vi "BlueSimpleReachTask.vi"() -> ()   [LabVIEW 2010]
uses:
  Controls/Bits to Write.ctl
panel:
  in  "Catch probability":i32 min=0 max=100 step=1
  out "Catch Trial?":bool
  in  "Catch Trial":bool
  out "DO Task":refnum<k21>="BlueSimple_DO_All"
  out "DI Task":refnum<k21>="BlueSimple_DI"
  out "Exp correct":i32
  out "Record flag":bool
  in  "Recenter motor":bool
  in  "Override bumps":bool
  in  "Start bump timer?":bool
  in  "Trial type":u16(ring) items=["Allflash/sensory", "Precue/memory"]
  in  "DBS On?":bool
  in  "Home+target OK?":bool
  out "Exp reset":bool
  out "target set #":i32
  in  "duration (s)":dbl=0.18 format="%.4f"
  in  "Inter-pulse delay":cluster{"Fix":dbl, "Rnd":dbl}={"Fix"=0.0, "Rnd"=1.5} {"Rnd" format="%.4f"; "Fix" format="%_4g"}
  in  "Autofeed?":bool
  out "Just initialized\nhold loop?":bool
  in  "Home reward?":bool
  in  "Home reward":cluster{"Fix":dbl, "Rnd":dbl} {"Rnd" format="%.4f"; "Fix" format="%_4g"}
  in  "Override 4":bool caption="Override 1"
  in  "Override 3":bool caption="Override 1"
  in  "Override 2":bool=TRUE caption="Override 1"
  in  "Override 1":bool=TRUE
  in  "LED lines":T1={"LED1"=1, "LED2"=2, "LED3"=3, "LED4"=4}
  in  "LED1":i16=5
  in  "LED2":i16=6
  in  "LED3":i16=7
  in  "LED4":i16=8
  in  "Bump Parameters":T2={"Distance (deg)"=2.0, "Travel time (ms)"=500.0} {"Travel time (ms)" min=0.1 max=10000.0; "Distance (deg)" min=0.1}
  in  "Bump delay":cluster{"Fix":dbl, "Rnd":dbl}={"Fix"=2.0, "Rnd"=8.0} {"Rnd" format="%.4f"; "Fix" format="%_4g"}
  in  "Sine parameters":T3={"Frequency"=1.0, "Degrees\npk-pk"=8.0, "Cycles"=10000} {"Degrees\npk-pk" min=0.1 max=120.0; "Frequency" min=0.001 format="%#_4g"}
  in  "Home":bool
  in  "Bumps":bool
  in  "Sines?":bool
  out "target set size":i32
  out "# target sets":u16
  in  "# Cycles":i16=20
  out "Instruct duration":dbl format="%.4f"
  out "Pre-I hold":dbl format="%.4f"
  out "Touching target\nlast time?":bool
  in  "Rand/Seq?":bool=TRUE
  in  "Target set":i16[](array[ring]) items=["1", "2", "3", "4"]
  in  "Block":T4(array[cluster])=array[6501 elements]
  in  "Settings In":T5={"Pre-I hold"={"Fixed (s)"=0.5, "Random (s)"=0.5}, "LED I duration"={"Fixed (s)"=0.5, "Random (s)"=0.0}, "All Flash?"=FALSE, "Pre-cue brightness"=0, "Post-I hold"={"Fixed (s)"=0.7, "Random (s)"=0.3}, "Post-I \nbounce-off"={"Fixed (s)"=0.3, "Random (s)"=0.0}, "Capture timeout"={"Fixed (s)"=1.5, "Random (s)"=0.0}, "Tone duration"={"Fixed (s)"=0.5, "Random (s)"=0.0}, "LED C duration"={"Fixed (s)"=0.5, "Random (s)"=0.0}, "Cue brightness"=0, "Hold duration"={"Fixed (s)"=0.3, "Random (s)"=0.0}, "Allowed\nbounce-off"={"Fixed (s)"=0.2, "Random (s)"=0.0}, "Post-capture brightness"=0, "Reward duration"={"Fixed (s)"=0.7, "Random (s)"=0.0}, "Intertrial interval"={"Fixed (s)"=0.5, "Random (s)"=0.0}, "Persistent Mode?"=FALSE, "Error bong?"=TRUE, "Critter"=0, "Blocks"=[], "Target set"=[], "Rand/Seq?"=TRUE, "Trial type"=0, "Sines?"=FALSE, "Bumps"=FALSE, "Sine parameters"={"Frequency"=0.25, "Degrees\npk-pk"=6.0, "Cycles"=10000}, "Bump timing"={"Fix"=2.0, "Rnd"=8.0}, "Bump Parameters"={"Distance (deg)"=2.0, "Travel time (ms)"=500.0}, "DBS On?"=FALSE, "Home reward?"=FALSE, "Home+target OK?"=FALSE} {"Bump Parameters"."Travel time (ms)" min=0.1 max=10000.0; "Bump Parameters"."Distance (deg)" min=0.1; "Bump timing"."Rnd" format="%.4f"; "Bump timing"."Fix" format="%_4g"; "Sine parameters"."Degrees\npk-pk" min=0.1 max=120.0; "Sine parameters"."Frequency" min=0.001 format="%#_4g"; "Trial type" items=["Allflash/sensory", "Precue/memory"]; "Target set" items=["1", "2", "3", "4"]; "Critter" items=["Mojo", "Smokey"]; "Post-I \nbounce-off"."Random (s)" format="%.4f"; "Post-I \nbounce-off"."Fixed (s)" format="%_4g"; "Allowed\nbounce-off"."Random (s)" format="%.4f"; "Allowed\nbounce-off"."Fixed (s)" format="%_4g"; "LED C duration"."Random (s)" format="%.4f"; "LED C duration"."Fixed (s)" format="%.4f"; "Capture timeout"."Random (s)" format="%.4f"; "Capture timeout"."Fixed (s)" format="%.4f"; "Post-I hold"."Random (s)" format="%.4f"; "Post-I hold"."Fixed (s)" format="%.4f"; "Hold duration"."Random (s)" format="%.4f"; "Hold duration"."Fixed (s)" format="%_4g"; "Intertrial interval"."Random (s)" format="%.4f"; "Intertrial interval"."Fixed (s)" format="%.4f"; "Reward duration"."Random (s)" format="%.4f"; "Reward duration"."Fixed (s)" format="%.4f"; "LED I duration"."Random (s)" format="%.4f"; "LED I duration"."Fixed (s)" format="%.4f"; "Tone duration"."Random (s)" format="%.4f"; "Tone duration"."Fixed (s)" format="%.4f"; "Pre-I hold"."Random (s)" format="%.4f"; "Pre-I hold"."Fixed (s)" format="%_4g"}
  in  "pause":bool
  out "Assign settings":bool
  out "current path":path
  out "next trial path":path
  in  "Critter":u16(ring) items=["Mojo", "Smokey", "Blue", "Odo", "Monk 5", "Monk 6", "Monk 7", "Monk 8", "Monk 9", "Monk 10"]
  out "Total incorrect":i32
  in  "Write Settings":bool
  in  "Read Settings":bool
  in  "All Flash?":bool
  in  "Post-capture brightness":i16 caption="Brightness"
  in  "Cue brightness":i16=6 caption="Brightness"
  in  "Pre-cue brightness":i16 caption="Brightness"
  out "Total correct":i32
  out "Total %":dbl
  out "Total trials":i32
  in  "Error\nbong?":bool=TRUE
  out "TS Home":bool
  out "TS 4":bool
  out "TS 3":bool
  out "TS 2":bool
  out "TS 1":bool
  out "Waveform Chart":T6(graph)
  out "Block trials":i32
  out "Block %":dbl
  in  "Reset\ncounters":bool
  in  "Post-I \nbounce-off":cluster{"Fix":dbl, "Rnd":dbl}={"Fix"=0.3, "Rnd"=0.0} caption="Allowed\nbounce-off" {"Rnd" format="%.4f"; "Fix" format="%_4g"}
  out "Exp trials":i32
  out "Exp %":dbl
  in  "Touch lines":T7={"Home touch"=0, "Touch 1"=1, "Touch 2"=2, "Touch 3"=3, "Touch 4"=4}
  out "Current stage":T8(ring)
  in  "Allowed\nbounce-off":cluster{"Fix":dbl, "Rnd":dbl}={"Fix"=0.2, "Rnd"=0.0} {"Rnd" format="%.4f"; "Fix" format="%_4g"}
  in  "LED C duration":cluster{"Fix":dbl, "Rnd":dbl}={"Fix"=0.5, "Rnd"=0.0} caption="LED duration" {"Rnd" format="%.4f"; "Fix" format="%.4f"}
  in  "Capture timeout":cluster{"Fix":dbl, "Rnd":dbl}={"Fix"=1.5, "Rnd"=0.0} caption="Response time" {"Rnd" format="%.4f"; "Fix" format="%.4f"}
  in  "Post-I hold":cluster{"Fix":dbl, "Rnd":dbl}={"Fix"=0.5, "Rnd"=0.5} {"Rnd" format="%.4f"; "Fix" format="%.4f"}
  out "Last trial successful?":bool
  in  "Persistent\n Mode?":bool
  in  "Touch 4":i16=4
  in  "Touch 3":i16=3
  in  "Touch 2":i16=2
  in  "Touch 1":i16=1
  in  "Home touch":i16
  in  "Hold duration":cluster{"Fix":dbl, "Rnd":dbl}={"Fix"=0.3, "Rnd"=0.0} {"Rnd" format="%.4f"; "Fix" format="%_4g"}
  out "Target":i16
  in  "stop":bool
  in  "device":i16=1
  in  "line direction map":i32=2147483616 format="%.0b"
  out "DIGIO task ID":u32 format="%.0x"
  out "error out":errorcluster
  in  "Intertrial interval":cluster{"Fix":dbl, "Rnd":dbl}={"Fix"=0.5, "Rnd"=0.0} {"Rnd" format="%.4f"; "Fix" format="%.4f"}
  in  "Reward duration":cluster{"Fix":dbl, "Rnd":dbl}={"Fix"=0.7, "Rnd"=0.0} {"Rnd" format="%.4f"; "Fix" format="%.4f"}
  in  "LED I duration":cluster{"Fix":dbl, "Rnd":dbl}={"Fix"=0.5, "Rnd"=0.0} caption="LED duration" {"Rnd" format="%.4f"; "Fix" format="%.4f"}
  in  "Tone duration":cluster{"Fix":dbl, "Rnd":dbl}={"Fix"=0.5, "Rnd"=0.0} {"Rnd" format="%.4f"; "Fix" format="%.4f"}
  in  "Pre-I hold":cluster{"Fix":dbl, "Rnd":dbl}={"Fix"=0.5, "Rnd"=0.5} {"Rnd" format="%.4f"; "Fix" format="%_4g"}
  # "Auto-feed"
  # "DBS"
  # "Pre-\ninstruction\nhold"
  # "Post-\ninstruction\nhold"
  # "Instruction"
  # "Target capture"
  # "Target hold"
  # "Reward"
  # "Intertrial"
  # "Motor"
  # "Override"
  # "+"
  # "+"
  # "+"
  # "Pre-\ninstruction\nhold"
  # "Instruction"
  # "Post-\ninstruction\nhold"
  # "Target capture"
  # "Target hold"
  # "Reward"
  # "Intertrial"
  # "+"
  # "+"
  # "+"
  # "+"
  # "+"
  # "+"
  # "+"
  # "+"
  # "+"
  # "+"
  # "+"
  # "+"
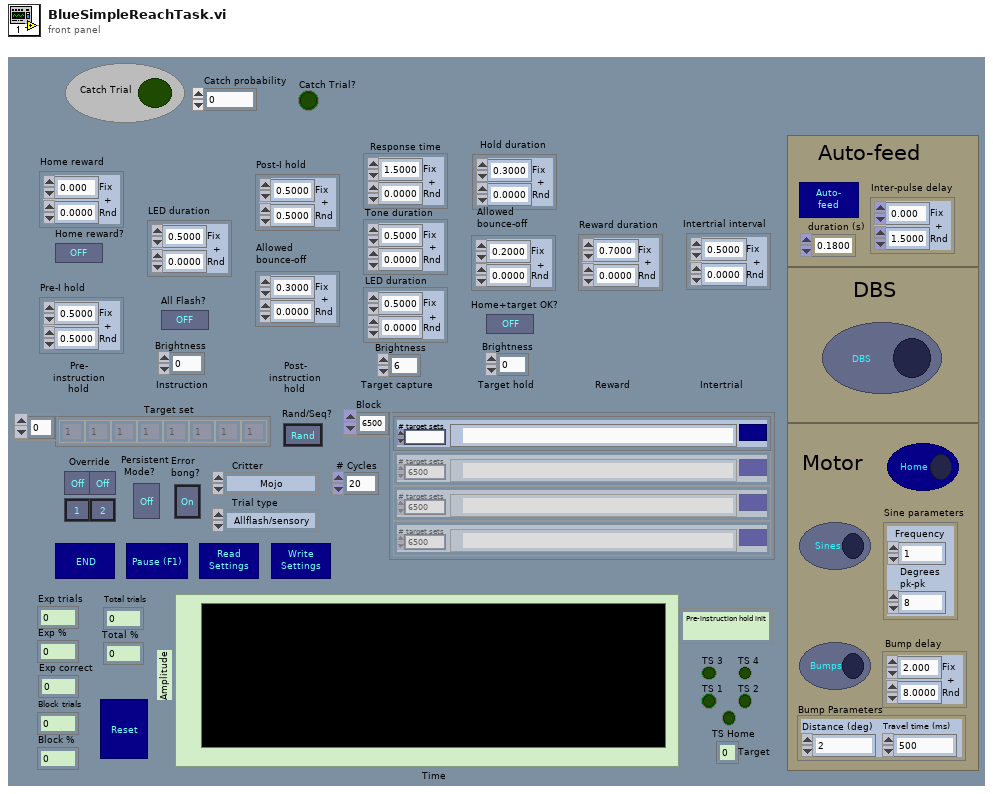
[diagram p1: front panel]
types:
  T1 = cluster{"LED1":i16, "LED2":i16, "LED3":i16, "LED4":i16}
  T2 = cluster{"Distance (deg)":dbl, "Travel time (ms)":dbl}
  T3 = cluster{"Frequency":dbl, "Degrees\npk-pk":dbl, "Cycles":i16}
  T4 = cluster{"Settings file":path, "# target sets":u16}[]
  T5 = cluster{"Pre-I hold":cluster{"Fixed (s)":dbl, "Random (s)":dbl}, "LED I duration":cluster{"Fixed (s)":dbl, "Random (s)":dbl}, "All Flash?":bool, "Pre-cue brightness":i16, "Post-I hold":cluster{"Fixed (s)":dbl, "Random (s)":dbl}, "Post-I \nbounce-off":cluster{"Fixed (s)":dbl, "Random (s)":dbl}, "Capture timeout":cluster{"Fixed (s)":dbl, "Random (s)":dbl}, "Tone duration":cluster{"Fixed (s)":dbl, "Random (s)":dbl}, "LED C duration":cluster{"Fixed (s)":dbl, "Random (s)":dbl}, "Cue brightness":i16, "Hold duration":cluster{"Fixed (s)":dbl, "Random (s)":dbl}, "Allowed\nbounce-off":cluster{"Fixed (s)":dbl, "Random (s)":dbl}, "Post-capture brightness":i16, "Reward duration":cluster{"Fixed (s)":dbl, "Random (s)":dbl}, "Intertrial interval":cluster{"Fixed (s)":dbl, "Random (s)":dbl}, "Persistent Mode?":bool, "Error bong?":bool, "Critter":u16, "Blocks":cluster{"Settings file":path, "# target sets":dbl}[], "Target set":i16[], "Rand/Seq?":bool, "Trial type":u16, "Sines?":bool, "Bumps":bool, "Sine parameters":cluster{"Frequency":dbl, "Degrees\npk-pk":dbl, "Cycles":i16}, "Bump timing":cluster{"Fix":dbl, "Rnd":dbl}, "Bump Parameters":cluster{"Distance (deg)":dbl, "Travel time (ms)":dbl}, "DBS On?":bool, "Home reward?":bool, "Home+target OK?":bool}
  T6 = cluster{"Segment Percentage":dbl, "Total % correct":dbl}
  T7 = cluster{"Home touch":i16, "Touch 1":i16, "Touch 2":i16, "Touch 3":i16, "Touch 4":i16}
  T8 = enum16{"Pre-instruction hold init", "Pre-instruction hold", "Instruction init", "Instruction", "Post-instruction hold init", "Post-instruction hold", "Target capture init", "Target capture", "Target hold init", "Target hold", "Reward stage", "Intertrial"}
  T9 = typedef "Bits to Write.ctl" = enum16{"LED 1 on", "LED 1 off", "LED 2 on", "LED 2 off", "LED 3 on", "LED 3 off", "LED 4 on", "LED 4 off", "All LEDs on", "All LEDs off", "In trial on", "In trial off", "Buzzer on", "Buzzer off", "Reward on", "Reward off", "Target number", "Trial type preQ on", "Trial type preQ off", "Error on", "Error off", "Trial number", "DBS on", "DBS off", "Sine on", "Sine off", "All Bits On", "All Bits Off", "Init", "Specify mask/pattern"}
  T10 = enum16{"Reset", "Increment", "Reset for exp", "Initialize"}
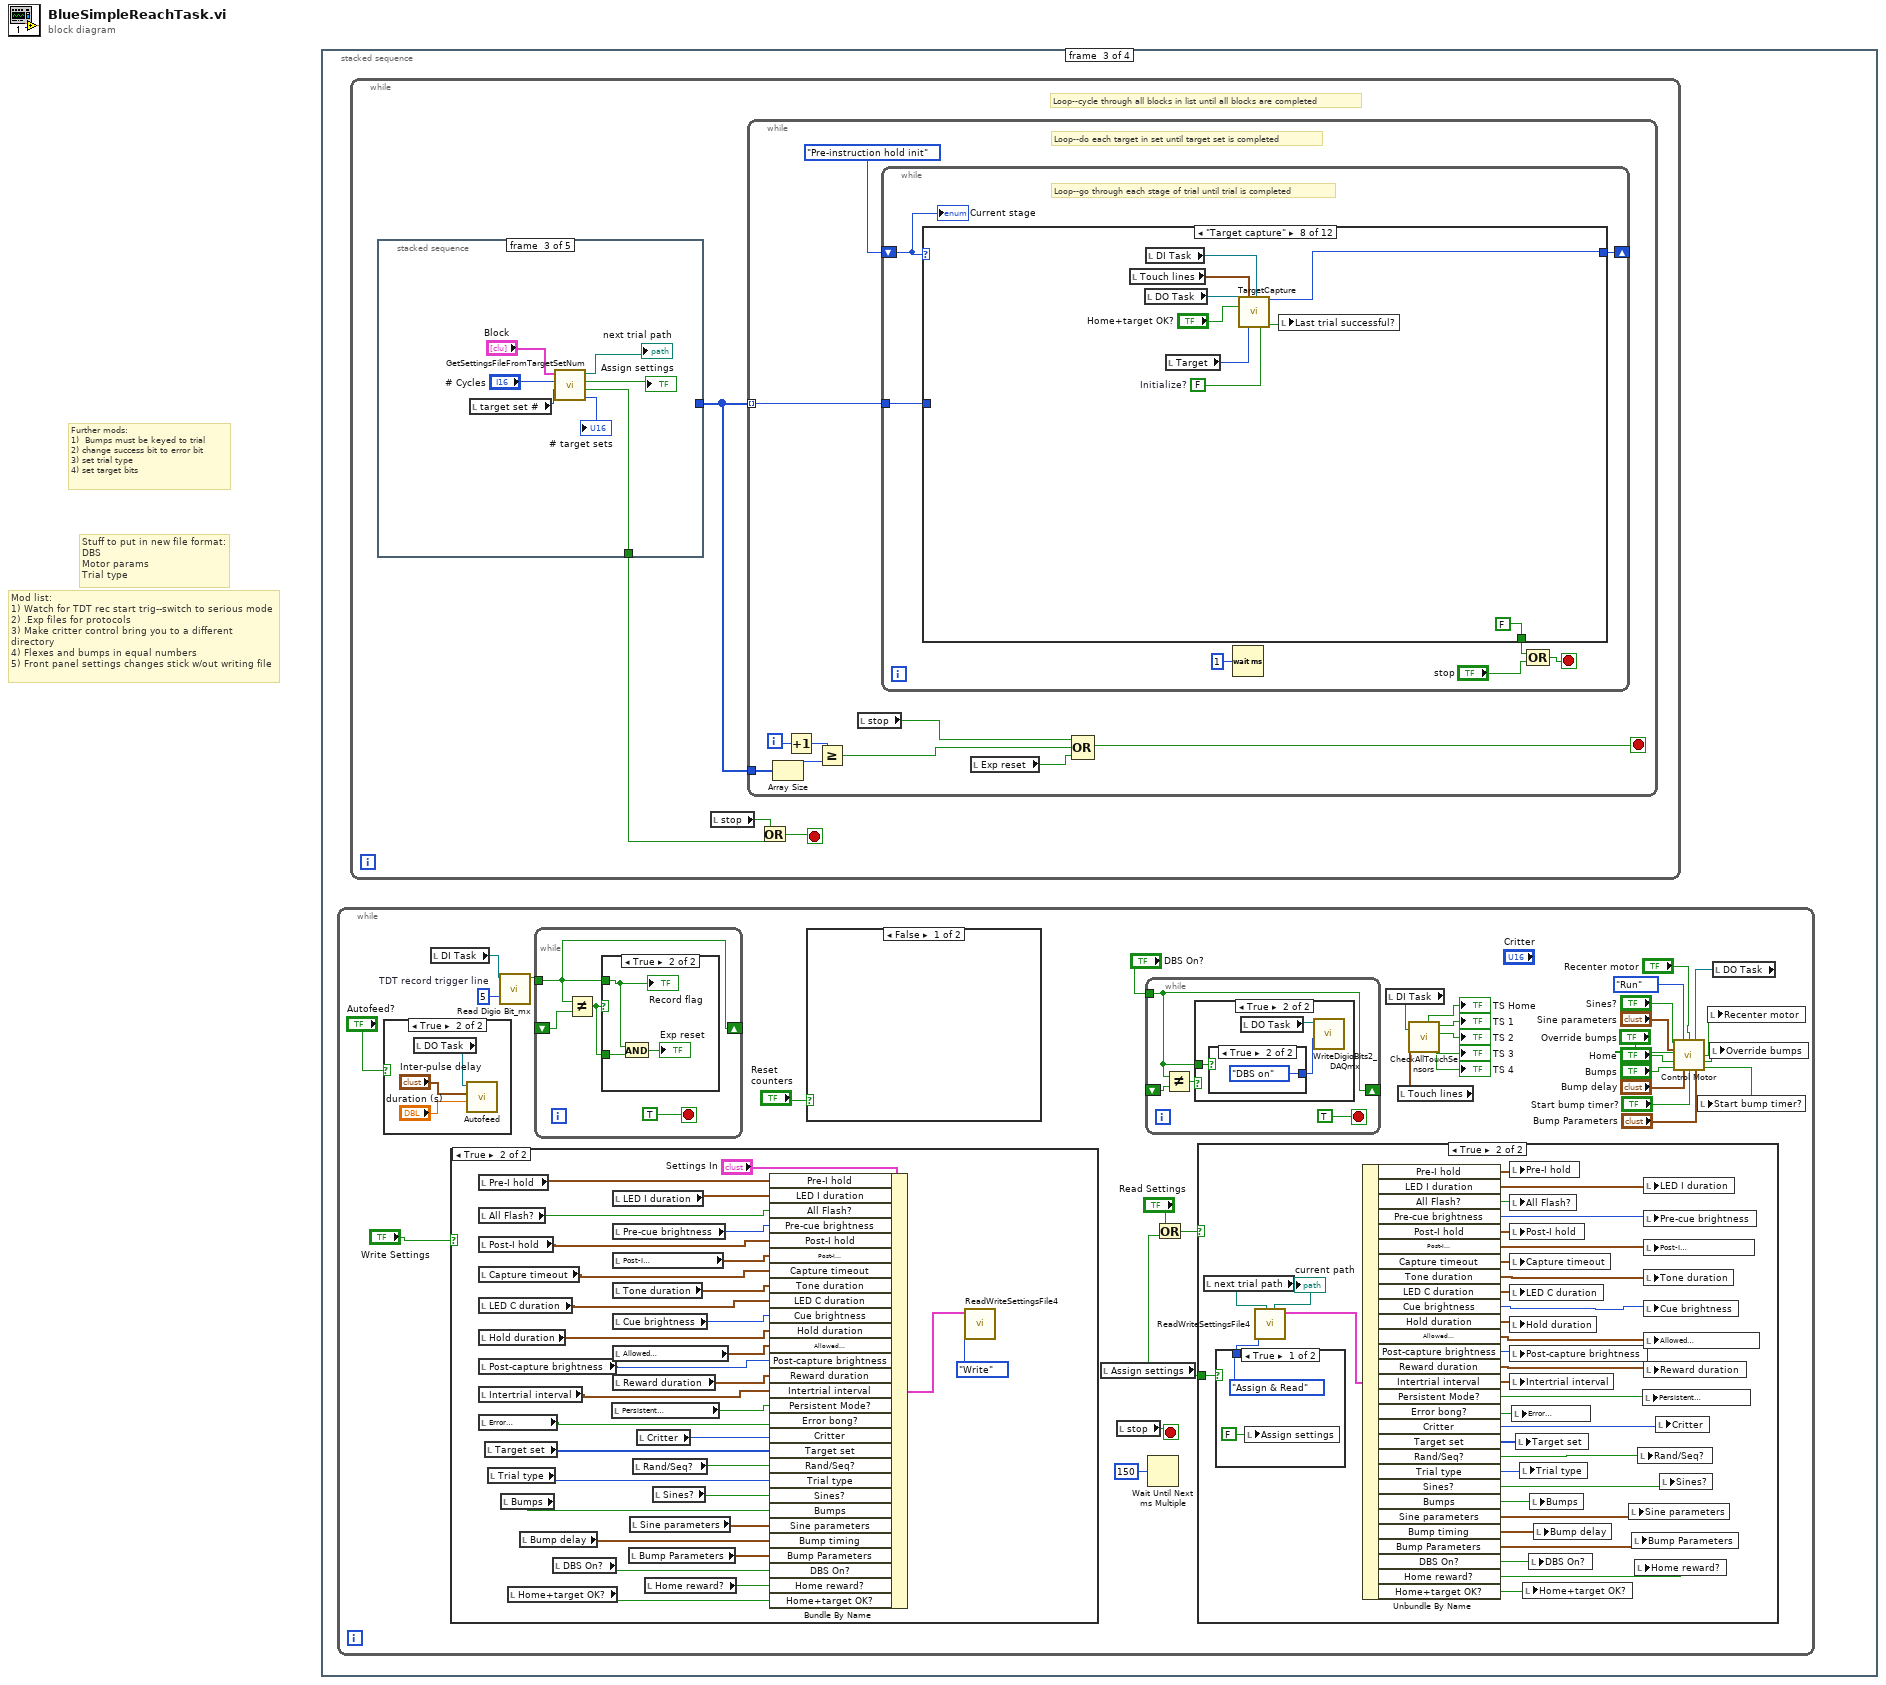
[diagram p0: block diagram]
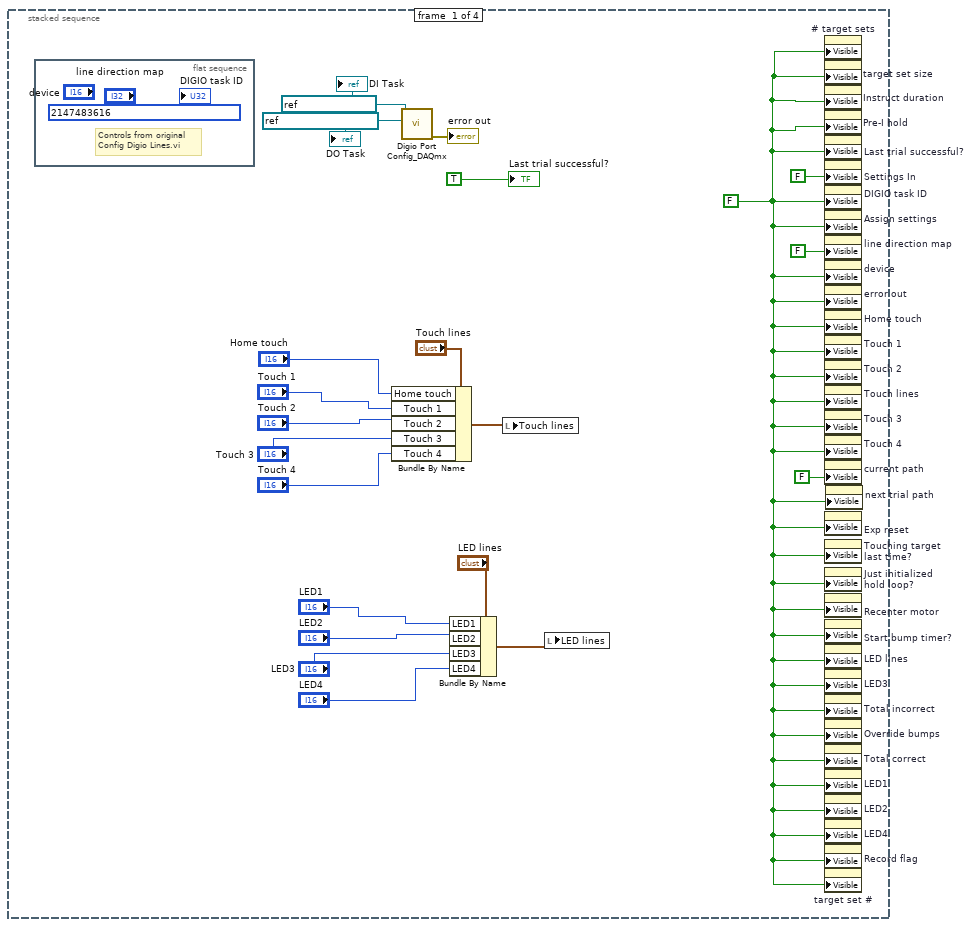
[diagram p2: hidden frame]
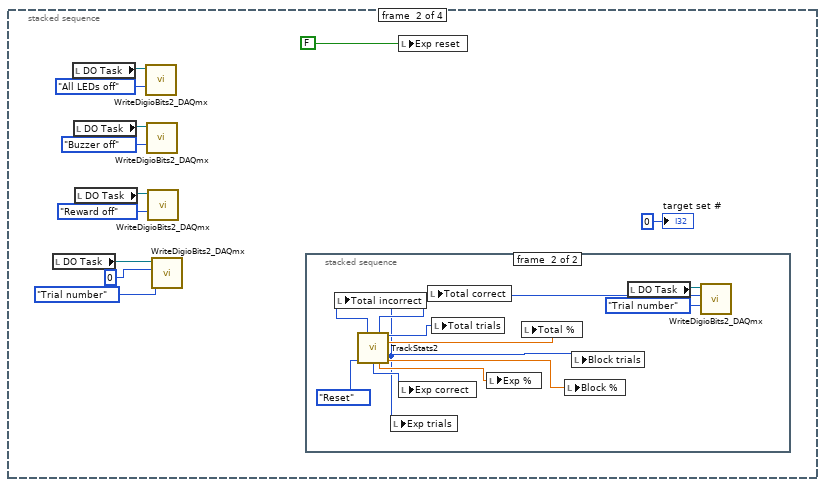
[diagram p3: hidden frame]
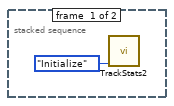
[diagram p4: hidden frame]
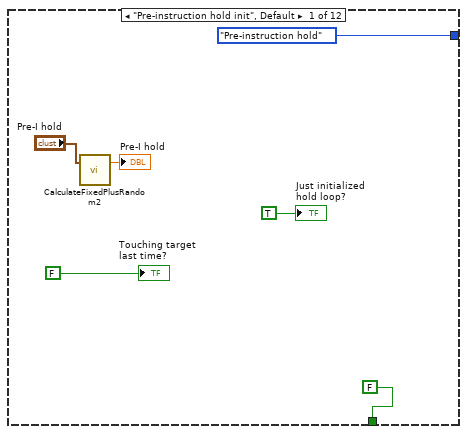
[diagram p5: hidden frame]
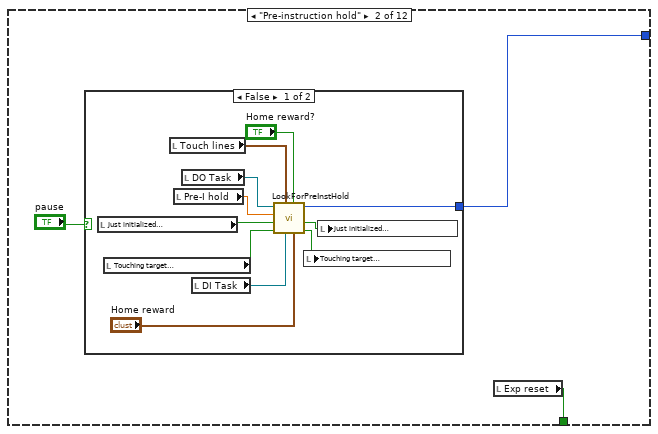
[diagram p6: hidden frame]
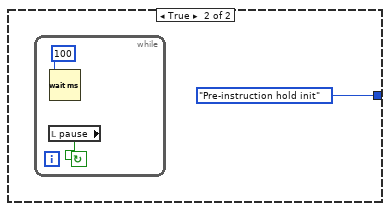
[diagram p7: hidden frame]
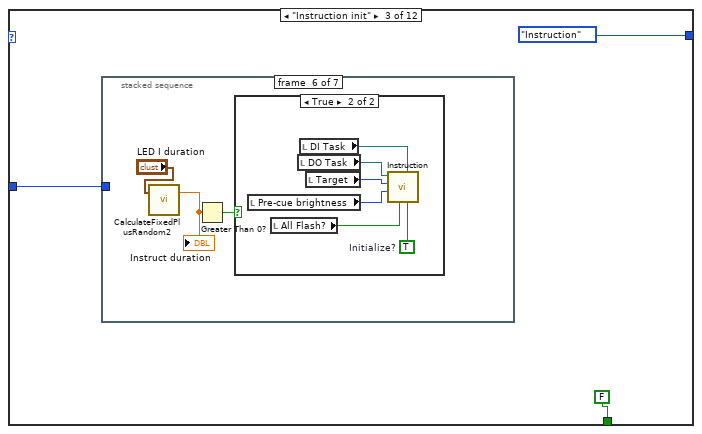
[diagram p8: hidden frame]
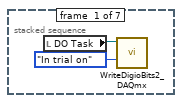
[diagram p9: hidden frame]
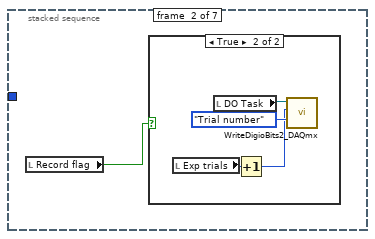
[diagram p10: hidden frame]
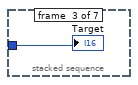
[diagram p12: hidden frame]
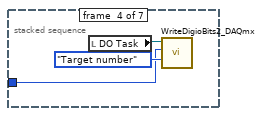
[diagram p13: hidden frame]
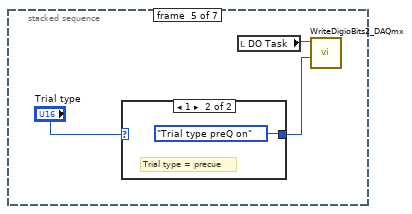
[diagram p14: hidden frame]
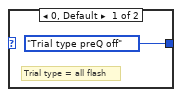
[diagram p15: hidden frame]
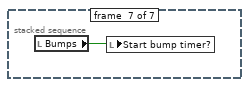
[diagram p17: hidden frame]
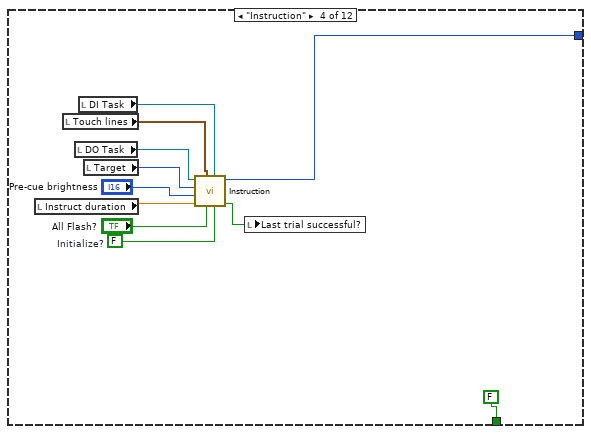
[diagram p18: hidden frame]
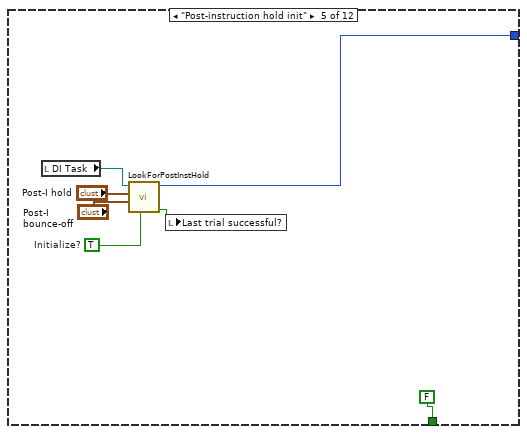
[diagram p19: hidden frame]
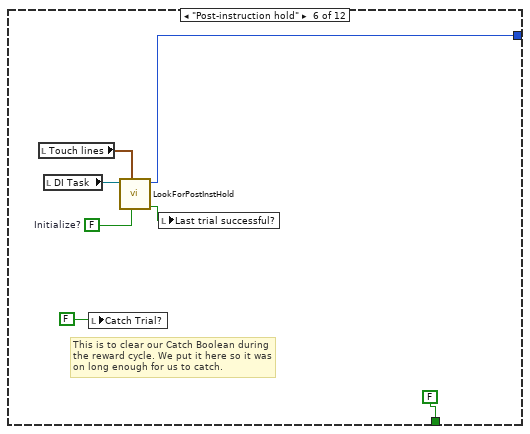
[diagram p20: hidden frame]
diagram:
  # "Stuff to put in new file format:\nDBS\nMotor params\nTrial type"
  # "Further mods:\n1)  Bumps must be keyed to trial\n2) change success bit to error bit\n3) set trial type\n4) set target bits"
  # "Mod list:\n1) Watch for TDT rec start trig--switch to serious mode\n2) .Exp files for protocols\n3) Make critter control bring you to a different directory\n4) Flexes and bumps in equal numbers\n5) Front panel settings changes stick w/out writing file"
  n1 = stacked-sequence {
    frame #0 {
      w2 = refnum<k21> "BlueSimple_DO_All" ("DO Task")
      w3 = refnum<k21> "BlueSimple_DI" ("DI Task")
      w4 = FALSE ("Persistent Mode?")
      n2 = flat-sequence {
        frame #0 {
          (unwired) 2147483616 ("line direction map")
          # "Controls from original\nConfig Digio Lines.vi"
        }
      }
      n3 = Bundle By Name(cluster="Touch lines", "Home touch"="Home touch", "Touch 1"="Touch 1", "Touch 2"="Touch 2", "Touch 3"="Touch 3", "Touch 4"="Touch 4") -> (w20:T7)
      n4 = call "Digio Port Config_DAQmx.vi"("DO Task"=w2, "DI Task"=w3) -> ("error out"=→"error out":errorcluster)  [unwired: 7 in]
      n5 = Bundle By Name(cluster="LED lines", "LED1"="LED1", "LED2"="LED2", "LED3"="LED3", "LED4"="LED4") -> (w8:T1)
      n6 = local write "Touch lines"(w20) -> ()
      n7 = local write "LED lines"(w8) -> ()
      n8 = property on="# target sets" class="DigNum (strict)"("Visible"=w4) -> ()  [unwired: 2 in, 2 out]
      n9 = property on="target set size" class="DigNum (strict)"("Visible"=w4) -> ()  [unwired: 2 in, 2 out]
      n10 = property on="Instruct duration" class="DigNum (strict)"("Visible"=w4) -> ()  [unwired: 2 in, 2 out]
      n11 = property on="Pre-I hold" class="DigNum (strict)"("Visible"=w4) -> ()  [unwired: 2 in, 2 out]
      n12 = property on="Last trial successful?" class="Bool (strict)"("Visible"=w4) -> ()  [unwired: 2 in, 2 out]
      n13 = property on="Settings In" class="Clust (strict)"("Visible"=FALSE) -> ()  [unwired: 2 in, 2 out]
      n14 = property on="DIGIO task ID" class="DigNum (strict)"("Visible"=w4) -> ()  [unwired: 2 in, 2 out]
      n15 = property on="Assign settings" class="Bool (strict)"("Visible"=w4) -> ()  [unwired: 2 in, 2 out]
      n16 = property on="line direction map" class="DigNum (strict)"("Visible"=FALSE) -> ()  [unwired: 2 in, 2 out]
      n17 = property on="device" class="DigNum (strict)"("Visible"=w4) -> ()  [unwired: 2 in, 2 out]
      n18 = property on="error out" class="Clust (strict)"("Visible"=w4) -> ()  [unwired: 2 in, 2 out]
      n19 = property on="Home touch" class="DigNum (strict)"("Visible"=w4) -> ()  [unwired: 2 in, 2 out]
      n20 = property on="Touch 1" class="DigNum (strict)"("Visible"=w4) -> ()  [unwired: 2 in, 2 out]
      n21 = property on="Touch 2" class="DigNum (strict)"("Visible"=w4) -> ()  [unwired: 2 in, 2 out]
      n22 = property on="Touch lines" class="Clust (strict)"("Visible"=w4) -> ()  [unwired: 2 in, 2 out]
      n23 = property on="Touch 3" class="DigNum (strict)"("Visible"=w4) -> ()  [unwired: 2 in, 2 out]
      n24 = property on="Touch 4" class="DigNum (strict)"("Visible"=w4) -> ()  [unwired: 2 in, 2 out]
      n25 = property on="current path" class="Path"("Visible"=FALSE) -> ()  [unwired: 2 in, 2 out]
      n26 = property on="Exp reset" class="Bool (strict)"("Visible"=w4) -> ()  [unwired: 2 in, 2 out]
      n27 = property on="Touching target\nlast time?" class="Bool (strict)"("Visible"=w4) -> ()  [unwired: 2 in, 2 out]
      n28 = property on="Just initialized\nhold loop?" class="Bool (strict)"("Visible"=w4) -> ()  [unwired: 2 in, 2 out]
      n29 = property on="Recenter motor" class="Bool (strict)"("Visible"=w4) -> ()  [unwired: 2 in, 2 out]
      n30 = property on="Start bump timer?" class="Bool (strict)"("Visible"=w4) -> ()  [unwired: 2 in, 2 out]
      n31 = property on="LED lines" class="Clust (strict)"("Visible"=w4) -> ()  [unwired: 2 in, 2 out]
      n32 = property on="LED3" class="DigNum (strict)"("Visible"=w4) -> ()  [unwired: 2 in, 2 out]
      n33 = property on="Total incorrect" class="DigNum (strict)"("Visible"=w4) -> ()  [unwired: 2 in, 2 out]
      n34 = property on="Override bumps" class="Bool (strict)"("Visible"=w4) -> ()  [unwired: 2 in, 2 out]
      n35 = property on="Total correct" class="DigNum (strict)"("Visible"=w4) -> ()  [unwired: 2 in, 2 out]
      n36 = property on="LED1" class="DigNum (strict)"("Visible"=w4) -> ()  [unwired: 2 in, 2 out]
      n37 = property on="LED2" class="DigNum (strict)"("Visible"=w4) -> ()  [unwired: 2 in, 2 out]
      n38 = property on="LED4" class="DigNum (strict)"("Visible"=w4) -> ()  [unwired: 2 in, 2 out]
      n39 = property on="Record flag" class="Bool (strict)"("Visible"=w4) -> ()  [unwired: 2 in, 2 out]
      n40 = property on="target set #" class="DigNum (strict)"("Visible"=w4) -> ()  [unwired: 2 in, 2 out]
      n41 = property on="next trial path" class="Path"("Visible"=w4) -> ()  [unwired: 2 in, 2 out]
      "Last trial successful?" <- TRUE ("Persistent Mode?")
      "DI Task" <- w3
      "DO Task" <- w2
    }
    frame #1 {
      n42 = local read "DO Task"() -> (w30:refnum<k21>)
      n43 = local read "DO Task"() -> (w23:refnum<k21>)
      n44 = local read "DO Task"() -> (w24:refnum<k21>)
      n45 = local read "DO Task"() -> (w26:refnum<k21>)
      n46 = call "WriteDigioBits2_DAQmx.vi"("Bits to write"=Bits_to_Write."All LEDs off", "DO Task"=w23) -> ()  [unwired: 9 in, 1 out]
      n47 = call "WriteDigioBits2_DAQmx.vi"("Bits to write"=Bits_to_Write."Buzzer off", "DO Task"=w24) -> ()  [unwired: 9 in, 1 out]
      n48 = call "WriteDigioBits2_DAQmx.vi"("Bits to write"=Bits_to_Write."Reward off", "DO Task"=w26) -> ()  [unwired: 9 in, 1 out]
      n49 = call "WriteDigioBits2_DAQmx.vi"("Bits to write"=Bits_to_Write."Trial number", "Number"=u32 0, "DO Task"=w30) -> ()  [unwired: 8 in, 1 out]
      n50 = stacked-sequence {
        frame #0 {
          n51 = call "TrackStats2.vi"("Command"=T10."Initialize") -> ()  [unwired: 6 in, 9 out]
        }
        frame #1 {
          n52 = call "TrackStats2.vi"("Command"=T10."Reset") -> ("Total incorrect"=w45:i32, "Total correct"=w44:i32, "# total trials"=w43:i32, "Total % correct"=w42:dbl, "Segment trials"=w38:i32, "Experiment trials"=w34:i32, "Experiment correct"=w37:i32, "Experiment %"=w40:dbl, "Segment Percentage"=w41:dbl)  [unwired: 6 in]
          n53 = local write "Total incorrect"(w45) -> ()
          n54 = local write "Exp trials"(w34) -> ()
          n55 = local write "Exp correct"(w37) -> ()
          n56 = local write "Total correct"(w44) -> ()
          n57 = local write "Total trials"(w43) -> ()
          n58 = local write "Exp %"(w40) -> ()
          n59 = local write "Total %"(w42) -> ()
          n60 = local write "Block %"(w41) -> ()
          n61 = local write "Block trials"(w38) -> ()
          n62 = local read "DO Task"() -> (w36:refnum<k21>)
          n63 = call "WriteDigioBits2_DAQmx.vi"("Bits to write"=Bits_to_Write."Trial number", "Number"=w34, "DO Task"=w36) -> ()  [unwired: 8 in, 1 out]
        }
      }
      n64 = local write "Exp reset"(FALSE ("Exp reset")) -> ()
      "target set #" <- 0 ("target set #")
    }
    frame #2 {
      n65 = while {
        stop <- w305 stop-if-true
        w275 = i16 5  # TDT record trigger line
        n66 = case shown="True" "Autofeed?" {
          frame False {
          }
          frame True {
            n67 = local read "DO Task"() -> (w315:refnum<k21>)
            n68 = call "Autofeed.vi"("duration"="duration (s)", "Auto-feed"="Inter-pulse delay", "DO Task"=w315) -> ()  [unwired: 4 in]
          }
        }
        n69 = local read "DI Task"() -> (w274:refnum<k21>)
        n70 = case shown="True" "Write Settings" {
          frame False {
          }
          frame True {
            n71 = local read "Pre-I hold"() -> (w356:cluster{"Fix":dbl, "Rnd":dbl})
            n72 = local read "All Flash?"() -> (w354:bool)
            n73 = local read "Post-I hold"() -> (w352:cluster{"Fix":dbl, "Rnd":dbl})
            n74 = local read "Capture timeout"() -> (w350:cluster{"Fix":dbl, "Rnd":dbl})
            n75 = local read "LED C duration"() -> (w348:cluster{"Fix":dbl, "Rnd":dbl})
            n76 = local read "Hold duration"() -> (w346:cluster{"Fix":dbl, "Rnd":dbl})
            n77 = local read "Post-capture brightness"() -> (w344:i16)
            n78 = local read "Intertrial interval"() -> (w342:cluster{"Fix":dbl, "Rnd":dbl})
            n79 = local read "Error\nbong?"() -> (w340:bool)
            n80 = local read "Target set"() -> (w336:i16[])
            n81 = local read "Trial type"() -> (w333:u16)
            n82 = local read "Bumps"() -> (w331:bool)
            n83 = local read "Home+target OK?"() -> (w325:bool)
            n84 = local read "Bump delay"() -> (w329:cluster{"Fix":dbl, "Rnd":dbl})
            n85 = local read "DBS On?"() -> (w327:bool)
            n86 = local read "Persistent\n Mode?"() -> (w341:bool)
            n87 = local read "LED I duration"() -> (w355:cluster{"Fix":dbl, "Rnd":dbl})
            n88 = local read "Pre-cue brightness"() -> (w353:i16)
            n89 = local read "Post-I \nbounce-off"() -> (w351:cluster{"Fix":dbl, "Rnd":dbl})
            n90 = local read "Tone duration"() -> (w349:cluster{"Fix":dbl, "Rnd":dbl})
            n91 = local read "Cue brightness"() -> (w347:i16)
            n92 = local read "Allowed\nbounce-off"() -> (w345:cluster{"Fix":dbl, "Rnd":dbl})
            n93 = local read "Reward duration"() -> (w343:cluster{"Fix":dbl, "Rnd":dbl})
            n94 = local read "Bump Parameters"() -> (w328:T2)
            n95 = local read "Sine parameters"() -> (w330:T3)
            n96 = local read "Rand/Seq?"() -> (w335:bool)
            n97 = local read "Critter"() -> (w337:u16)
            n98 = local read "Home reward?"() -> (w326:bool)
            n99 = local read "Sines?"() -> (w332:bool)
            n100 = Bundle By Name(cluster="Settings In", "Pre-I hold"=w356, "LED I duration"=w355, "All Flash?"=w354, "Pre-cue brightness"=w353, "Post-I hold"=w352, "Post-I \nbounce-off"=w351, "Capture timeout"=w350, "Tone duration"=w349, "LED C duration"=w348, "Cue brightness"=w347, "Hold duration"=w346, "Allowed\nbounce-off"=w345, "Post-capture brightness"=w344, "Reward duration"=w343, "Intertrial interval"=w342, "Persistent Mode?"=w341, "Error bong?"=w340, "Critter"=w337, "Target set"=w336, "Rand/Seq?"=w335, "Trial type"=w333, "Sines?"=w332, "Bumps"=w331, "Sine parameters"=w330, "Bump timing"=w329, "Bump Parameters"=w328, "DBS On?"=w327, "Home reward?"=w326, "Home+target OK?"=w325) -> (w334:T5)
            n101 = call "ReadWriteSettingsFile4.vi"("Read/write"=enum16{"Query & Read", "Assign & Read", "Write"}."Write", "Settings In"=w334) -> ()  [unwired: 4 in, 4 out]
          }
        }
        n102 = call "Read Digio Bit_mx.vi"("line"=w275, "DI Task"=w274) -> ("line state"=w273:bool)  [unwired: 7 in, 1 out]
        n103 = while {
          tunnel: w273 -> [w319]
          shift-right: [w319] -> _
          shift-left: _ -> [w320]
          stop <- TRUE stop-if-true
          n104 = Not Equal?(x=w319, y=w320) -> (x != y?=w318:bool)
          n105 = case shown="True" w318 {
            tunnel: w319 -> [_ w322]
            tunnel: w318 -> [_ w323]
            frame False {
            }
            frame True {
              n106 = And(x=w322, y=w323) -> (x .and. y?=→"Exp reset":bool)
              "Record flag" <- w322
            }
          }
        }
        n107 = case shown="False" "Reset\ncounters" {
          frame False {
          }
          frame True {
            n108 = call "TrackStats2.vi"("Command"=T10."Reset") -> ("Total incorrect"=w402:i32, "Total correct"=w401:i32, "# total trials"=w400:i32, "Total % correct"=w399:dbl, "Segment trials"=w398:i32, "Experiment trials"=w395:i32, "Experiment %"=w396:dbl, "Segment Percentage"=w397:dbl)  [unwired: 6 in, 1 out]
            n109 = local write "Total incorrect"(w402) -> ()
            n110 = local write "Total correct"(w401) -> ()
            n111 = local write "Exp trials"(w395) -> ()
            n112 = local write "Exp %"(w396) -> ()
            n113 = local write "Block %"(w397) -> ()
            n114 = local write "Block trials"(w398) -> ()
            n115 = local write "Total trials"(w400) -> ()
            n116 = local write "Total %"(w399) -> ()
          }
        }
        n117 = local read "Assign settings"() -> (w293:bool)
        n118 = local read "stop"() -> (w305:bool)
        n119 = while {
          shift-right: [w307] -> _
          shift-left: _ -> [w308]
          tunnel: "DBS On?" -> [w307]
          stop <- TRUE stop-if-true
          n120 = Not Equal?(x=w307, y=w308) -> (x != y?=w306:bool)
          n121 = case shown="True" w306 {
            tunnel: w307 -> [_ w312]
            frame False {
            }
            frame True {
              n122 = case shown="True" w312 {
                tunnel: [Bits_to_Write."DBS off" ("Bits to write") Bits_to_Write."DBS on" ("Bits to write")] -> w310
                frame False {
                }
                frame True {
                }
              }
              n123 = local read "DO Task"() -> (w311:refnum<k21>)
              n124 = call "WriteDigioBits2_DAQmx.vi"("Bits to write"=w310, "DO Task"=w311) -> ()  [unwired: 9 in, 1 out]
            }
          }
        }
        n125 = Wait Until Next ms Multiple(millisecond multiple=u32 150) -> ()  [unwired: 1 out]
        n126 = Or(x="Read Settings", y=w293) -> (x .or. y?=w294:bool)
        n127 = case shown="True" w294 {
          tunnel: w293 -> [_ w369]
          frame False {
          }
          frame True {
            n128 = local read "next trial path"() -> (w370:path)
            n129 = case shown="True" w369 {
              tunnel: [enum16{"Query & Read", "Assign & Read", "Write"}."Assign & Read" ("Read/write") enum16{"Query & Read", "Assign & Read", "Write"}."Query & Read" ("Read/write")] -> w372
              frame True {
                n130 = local write "Assign settings"(FALSE ("Assign settings")) -> ()
              }
              frame False {
              }
            }
            n131 = call "ReadWriteSettingsFile4.vi"("file path"=w370, "Read/write"=w372) -> ("Settings Out"=w390:T5, "current path"=→"current path":path)  [unwired: 4 in, 2 out]
            n132 = Unbundle By Name(w390) -> ("Pre-I hold"=w389:cluster{"Fixed (s)":dbl, "Random (s)":dbl}, "LED I duration"=w388:cluster{"Fixed (s)":dbl, "Random (s)":dbl}, "All Flash?"=w387:bool, "Pre-cue brightness"=w386:i16, "Post-I hold"=w385:cluster{"Fixed (s)":dbl, "Random (s)":dbl}, "Post-I \nbounce-off"=w384:cluster{"Fixed (s)":dbl, "Random (s)":dbl}, "Capture timeout"=w383:cluster{"Fixed (s)":dbl, "Random (s)":dbl}, "Tone duration"=w382:cluster{"Fixed (s)":dbl, "Random (s)":dbl}, "LED C duration"=w381:cluster{"Fixed (s)":dbl, "Random (s)":dbl}, "Cue brightness"=w380:i16, "Hold duration"=w379:cluster{"Fixed (s)":dbl, "Random (s)":dbl}, "Allowed\nbounce-off"=w378:cluster{"Fixed (s)":dbl, "Random (s)":dbl}, "Post-capture brightness"=w377:i16, "Reward duration"=w376:cluster{"Fixed (s)":dbl, "Random (s)":dbl}, "Intertrial interval"=w375:cluster{"Fixed (s)":dbl, "Random (s)":dbl}, "Persistent Mode?"=w374:bool, "Error bong?"=w373:bool, "Critter"=w368:u16, "Target set"=w367:i16[], "Rand/Seq?"=w366:bool, "Trial type"=w365:u16, "Sines?"=w364:bool, "Bumps"=w363:bool, "Sine parameters"=w362:T3, "Bump timing"=w361:cluster{"Fix":dbl, "Rnd":dbl}, "Bump Parameters"=w360:T2, "DBS On?"=w359:bool, "Home reward?"=w358:bool, "Home+target OK?"=w357:bool)
            n133 = local write "Pre-I hold"(w389) -> ()
            n134 = local write "All Flash?"(w387) -> ()
            n135 = local write "Post-I hold"(w385) -> ()
            n136 = local write "Capture timeout"(w383) -> ()
            n137 = local write "LED C duration"(w381) -> ()
            n138 = local write "Hold duration"(w379) -> ()
            n139 = local write "Post-capture brightness"(w377) -> ()
            n140 = local write "Intertrial interval"(w375) -> ()
            n141 = local write "Error\nbong?"(w373) -> ()
            n142 = local write "Target set"(w367) -> ()
            n143 = local write "Trial type"(w365) -> ()
            n144 = local write "Home+target OK?"(w357) -> ()
            n145 = local write "DBS On?"(w359) -> ()
            n146 = local write "Bumps"(w363) -> ()
            n147 = local write "Bump delay"(w361) -> ()
            n148 = local write "Sine parameters"(w362) -> ()
            n149 = local write "Bump Parameters"(w360) -> ()
            n150 = local write "Home reward?"(w358) -> ()
            n151 = local write "Rand/Seq?"(w366) -> ()
            n152 = local write "Persistent\n Mode?"(w374) -> ()
            n153 = local write "LED I duration"(w388) -> ()
            n154 = local write "Pre-cue brightness"(w386) -> ()
            n155 = local write "Post-I \nbounce-off"(w384) -> ()
            n156 = local write "Tone duration"(w382) -> ()
            n157 = local write "Cue brightness"(w380) -> ()
            n158 = local write "Allowed\nbounce-off"(w378) -> ()
            n159 = local write "Reward duration"(w376) -> ()
            n160 = local write "Critter"(w368) -> ()
            n161 = local write "Sines?"(w364) -> ()
          }
        }
        n162 = local read "DI Task"() -> (w303:refnum<k21>)
        n163 = local read "Touch lines"() -> (w302:T7)
        n164 = call "CheckAllTouchSensors.vi"("Touch sensor lines"=w302, "DI Task"=w303) -> ("TS 4"=→"TS 4":bool, "TS 3"=→"TS 3":bool, "TS 2"=→"TS 2":bool, "TS 1"=→"TS 1":bool, "Home?"=→"TS Home":bool)
        n165 = local read "DO Task"() -> (w276:refnum<k21>)
        n166 = call "Control Motor.vi"("Sines?"="Sines?", "Command"=enum16{"Initialize", "Home", "Run", "Disable"}."Run", "Re-center\nmotor"="Recenter motor", "DO Task"=w276, "Sine parameters"="Sine parameters", "Override bumps"="Override bumps", "Home"="Home", "Bumps"="Bumps", "Bump timing"="Bump delay", "Start bump timer?"="Start bump timer?", "Bump Parameters"="Bump Parameters") -> ("Reset\nrecenter"=w278:bool, "Reset override bumps"=w280:bool, "Reset start button"=w282:bool)  [unwired: 2 in]
        n167 = local write "Start bump timer?"(w282) -> ()
        n168 = local write "Recenter motor"(w278) -> ()
        n169 = local write "Override bumps"(w280) -> ()
      }
      n170 = while {
        stop <- w46 stop-if-true
        # "Loop--cycle through all blocks in list until all blocks are completed"
        n171 = stacked-sequence {
          tunnel: [_ _ _ _ w260] -> w49
          tunnel: [_ _ w252 _ _] -> w47
          frame #0 {
            n172 = local read "Exp reset"() -> (w235:bool)
            n173 = case shown="True" w235 {
              frame False {
              }
              frame True {
                n174 = stacked-sequence {
                  frame #0 {
                    n175 = call <vilib>:"Beep.vi"() -> ()  [unwired: 12 in]
                    n176 = Wait (ms)(milliseconds to wait=u32 5) -> ()  [unwired: 1 out]
                  }
                  frame #1 {
                    n177 = local write "Exp reset"(FALSE ("Exp reset")) -> ()
                  }
                  frame #2 {
                    n178 = local write "target set #"(0 ("target set #")) -> ()
                  }
                  frame #3 {
                    n179 = call "TrackStats2.vi"("Command"=T10."Reset for exp") -> ("Total incorrect"=w248:i32, "Total correct"=w247:i32, "# total trials"=w246:i32, "Total % correct"=w245:dbl, "Segment trials"=w244:i32, "Experiment trials"=w241:i32, "Experiment correct"=w239:i32, "Experiment %"=w242:dbl, "Segment Percentage"=w243:dbl)  [unwired: 6 in]
                    n180 = local write "Exp trials"(w241) -> ()
                    n181 = local write "Total incorrect"(w248) -> ()
                    n182 = local write "Total correct"(w247) -> ()
                    n183 = local write "Exp %"(w242) -> ()
                    n184 = local write "Exp correct"(w239) -> ()
                    n185 = local write "Block %"(w243) -> ()
                    n186 = local write "Block trials"(w244) -> ()
                    n187 = local write "Total trials"(w246) -> ()
                    n188 = local write "Total %"(w245) -> ()
                  }
                }
              }
            }
          }
          frame #1 {
            n189 = local read "target set #"() -> (w249:i32)
            n190 = Increment(x=w249) -> (x+1=w250:i32)
            n191 = local write "target set #"(w250) -> ()
          }
          frame #2 {
            n192 = local read "target set #"() -> (w257:i32)
            n193 = call "GetSettingsFileFromTargetSetNum.vi"("target set #"=w257, "# Cycles"="# Cycles", "Block"="Block") -> ("# target sets"=→"# target sets":u16, "Completed list?"=w252:bool, "apply new settings?"=→"Assign settings":bool, "Settings file"=→"next trial path":path)  [unwired: 1 in]
          }
          frame #3 {
            n194 = local read "Assign settings"() -> (w258:bool)
            n195 = case shown="True" w258 {
              frame False {
              }
              frame True {
                # "500ms delay to allow \nsettings loop below to\ninstantiate new settings"
                n196 = Wait (ms)(milliseconds to wait=u32 500) -> ()  [unwired: 1 out]
              }
            }
          }
          frame #4 {
            n197 = call "TargetOverride.vi"("Override 1"="Override 1", "Override 2"="Override 2", "Override 3"="Override 3", "Override 4"="Override 4", "Target set"="Target set") -> ("Target set out"=w266:i16[])  [unwired: 1 in]
            n198 = case shown="True" "Rand/Seq?" {
              tunnel: w266 -> [w270 w272]
              tunnel: [w270 w271] -> w261
              frame False {
              }
              frame True {
                n199 = call "RandomizeTargetSet.vi"("Target set"=w272) -> ("Target set rand order"=w271:i16[])
              }
            }
            n200 = Increment(x=w261) -> (x+1=w260:i16[])
            n201 = Array Size(array=w260) -> (size(s)=→"target set size":i32)
          }
        }
        n202 = local read "stop"() -> (w48:bool)
        n203 = while {
          tunnel: w49 -> [w58] mode=indexing
          tunnel: w49 -> [w57]
          i -> [w56]
          stop <- w50 stop-if-true
          # "Loop--do each target in set until target set is completed"
          n204 = Array Size(array=w57) -> (size(s)=w55:i32)
          n205 = Increment(x=w56) -> (x+1=w54:i32)
          n206 = Greater Or Equal?(x=w54, y=w55) -> (x >= y?=w52:bool)
          n207 = local read "stop"() -> (w53:bool)
          n208 = while {
            shift-right: [w66] -> _
            shift-left: T8."Pre-instruction hold init" ("Current stage") -> [w65]
            tunnel: w58 -> [w64]
            stop <- w61 stop-if-true
            # "Loop--go through each stage of trial until trial is completed"
            n209 = case shown="\"Target capture\"" w65 {
              tunnel: [T8."Pre-instruction hold" ("Current stage") w75 T8."Instruction" ("Current stage") w123 w131 w143 T8."Target capture" ("Current stage") w163 T8."Target hold" ("Current stage") w181 T8."Intertrial" ("Current stage") T8."Pre-instruction hold init" ("Current stage")] -> w66
              tunnel: [FALSE ("Just initialized\nhold loop?") w73 FALSE ("End of trial") FALSE ("End of trial") FALSE ("End of trial") FALSE ("End of trial") FALSE ("End of trial") FALSE ("End of trial") FALSE ("End of trial") FALSE ("End of trial") FALSE ("End of trial") w219] -> w63
              tunnel: w64 -> [_ _ w90 _ _ _ _ _ _ _ _ _]
              frame "Pre-instruction hold init", Default {
                n210 = call "CalculateFixedPlusRandom2.vi"("Component times"="Pre-I hold") -> ("Composite time"=→"Pre-I hold":dbl)  [unwired: 1 in, 1 out]
                "Touching target\nlast time?" <- FALSE ("Touching target\nlast time?")
                "Just initialized\nhold loop?" <- TRUE ("Just initialized\nhold loop?")
              }
              frame "Pre-instruction hold" {
                n211 = case shown="False" "pause" {
                  tunnel: [w86 T8."Pre-instruction hold init" ("Current stage")] -> w75
                  frame False {
                    n212 = local read "Just initialized\nhold loop?"() -> (w81:bool)
                    n213 = local read "Touching target\nlast time?"() -> (w83:bool)
                    n214 = local read "Touch lines"() -> (w84:T7)
                    n215 = local read "Pre-I hold"() -> (w85:dbl)
                    n216 = local read "DO Task"() -> (w77:refnum<k21>)
                    n217 = local read "DI Task"() -> (w76:refnum<k21>)
                    n218 = call "LookForPreInstHold.vi"("Home reward"="Home reward", "Home reward?"="Home reward?", "DI Task"=w76, "Touch lines"=w84, "Touching home\nlast time?"=w83, "Just initialized\nhold loop?"=w81, "Composite time"=w85, "DO Task"=w77) -> ("Touching home\nthis time?"=w82:bool, "Just initialized\nhold loop out?"=w80:bool, "Next stage in trial"=w86:T8)  [unwired: 1 in]
                    n219 = local write "Touching target\nlast time?"(w82) -> ()
                    n220 = local write "Just initialized\nhold loop?"(w80) -> ()
                  }
                  frame True {
                    n221 = while {
                      stop <- w88 continue-if-true
                      n222 = local read "pause"() -> (w88:bool)
                      n223 = Wait (ms)(milliseconds to wait=u32 100) -> ()  [unwired: 1 out]
                    }
                  }
                }
                n224 = local read "Exp reset"() -> (w73:bool)
              }
              frame "Instruction init" {
                n225 = stacked-sequence {
                  tunnel: w90 -> [_ _ w100 w101 _ _ _]
                  frame #0 {
                    n226 = local read "DO Task"() -> (w93:refnum<k21>)
                    n227 = call "WriteDigioBits2_DAQmx.vi"("Bits to write"=Bits_to_Write."In trial on", "DO Task"=w93) -> ()  [unwired: 9 in, 1 out]
                  }
                  frame #1 {
                    n228 = local read "Record flag"() -> (w95:bool)
                    n229 = case shown="True" w95 {
                      frame False {
                      }
                      frame True {
                        n230 = local read "Exp trials"() -> (w99:i32)
                        n231 = local read "DO Task"() -> (w97:refnum<k21>)
                        n232 = Increment(x=w99) -> (x+1=w96:i32)
                        n233 = call "WriteDigioBits2_DAQmx.vi"("Bits to write"=Bits_to_Write."Trial number", "Number"=w96, "DO Task"=w97) -> ()  [unwired: 8 in, 1 out]
                      }
                    }
                  }
                  frame #2 {
                    "Target" <- w100
                  }
                  frame #3 {
                    n234 = local read "DO Task"() -> (w102:refnum<k21>)
                    n235 = call "WriteDigioBits2_DAQmx.vi"("Bits to write"=Bits_to_Write."Target number", "Number"=w101, "DO Task"=w102) -> ()  [unwired: 8 in, 1 out]
                  }
                  frame #4 {
                    n236 = case shown="1" "Trial type" {
                      tunnel: [Bits_to_Write."Trial type preQ off" ("Bits to write") Bits_to_Write."Trial type preQ on" ("Bits to write")] -> w104
                      frame 0, Default {
                        # "Trial type = all flash"
                      }
                      frame 1 {
                        # "Trial type = precue"
                      }
                    }
                    n237 = local read "DO Task"() -> (w105:refnum<k21>)
                    n238 = call "WriteDigioBits2_DAQmx.vi"("Bits to write"=w104, "DO Task"=w105) -> ()  [unwired: 9 in, 1 out]
                  }
                  frame #5 {
                    n239 = call "CalculateFixedPlusRandom2.vi"("Component times"="LED I duration") -> ("Composite time"=w109:dbl)  [unwired: 1 in, 1 out]
                    "Instruct duration" <- w109
                    n240 = Greater Than 0?(x=w109) -> (x > 0?=w110:bool)
                    n241 = case shown="True" w110 {
                      frame False {
                      }
                      frame True {
                        w117 = TRUE  # Initialize?
                        n242 = local read "Pre-cue brightness"() -> (w115:i16)
                        n243 = local read "All Flash?"() -> (w114:bool)
                        n244 = local read "DO Task"() -> (w113:refnum<k21>)
                        n245 = local read "DI Task"() -> (w112:refnum<k21>)
                        n246 = local read "Target"() -> (w116:i16)
                        n247 = call "Instruction.vi"("Initialize?"=w117, "DI Task"=w112, "All Flash?"=w114, "brightness"=w115, "Target"=w116, "DO Task"=w113) -> ()  [unwired: 4 in, 2 out]
                      }
                    }
                  }
                  frame #6 {
                    n248 = local read "Bumps"() -> (w118:bool)
                    n249 = local write "Start bump timer?"(w118) -> ()
                  }
                }
              }
              frame "Instruction" {
                w128 = FALSE  # Initialize?
                n250 = local read "Instruct duration"() -> (w124:dbl)
                n251 = local read "Touch lines"() -> (w129:T7)
                n252 = local read "DO Task"() -> (w120:refnum<k21>)
                n253 = local read "DI Task"() -> (w119:refnum<k21>)
                n254 = local read "Target"() -> (w126:i16)
                n255 = call "Instruction.vi"("Initialize?"=w128, "DI Task"=w119, "All Flash?"="All Flash?", "Touch lines"=w129, "Instruction duration"=w124, "brightness"="Pre-cue brightness", "Target"=w126, "DO Task"=w120) -> ("Last trial successful?"=w127:bool, "Go to stage"=w123:T8)  [unwired: 2 in]
                n256 = local write "Last trial successful?"(w127) -> ()
              }
              frame "Post-instruction hold init" {
                w135 = TRUE  # Initialize?
                n257 = local read "DI Task"() -> (w136:refnum<k21>)
                n258 = call "LookForPostInstHold.vi"("Initialize?"=w135, "Post-I \nbounce-off"="Post-I \nbounce-off", "Post-I hold"="Post-I hold", "DI Task"=w136) -> ("Last trial successful?"=w134:bool, "Go to stage"=w131:T8)  [unwired: 6 in]
                n259 = local write "Last trial successful?"(w134) -> ()
              }
              frame "Post-instruction hold" {
                w140 = FALSE  # Initialize?
                # "This is to clear our Catch Boolean during\nthe reward cycle. We put it here so it was\non long enough for us to catch."
                n260 = local read "Touch lines"() -> (w142:T7)
                n261 = local read "DI Task"() -> (w141:refnum<k21>)
                n262 = local write "Catch Trial?"(FALSE) -> ()
                n263 = call "LookForPostInstHold.vi"("Initialize?"=w140, "Touch lines"=w142, "DI Task"=w141) -> ("Last trial successful?"=w139:bool, "Go to stage"=w143:T8)  [unwired: 7 in]
                n264 = local write "Last trial successful?"(w139) -> ()
              }
              frame "Target capture init" {
                w153 = TRUE  # Initialize?
                n265 = local read "DO Task"() -> (w145:refnum<k21>)
                n266 = local read "DI Task"() -> (w144:refnum<k21>)
                n267 = local read "Target"() -> (w151:i16)
                n268 = call "TargetCapture.vi"("DO Task"=w145, "DI Task"=w144, "Response time"="Capture timeout", "Tone duration"="Tone duration", "LED C duration"="LED C duration", "Target"=w151, "Cue brightness"="Cue brightness", "Initialize?"=w153) -> ("Last trial successful?"=w149:bool)  [unwired: 6 in, 1 out]
                n269 = local write "Last trial successful?"(w149) -> ()
              }
              frame "Target capture" {
                w159 = FALSE  # Initialize?
                n270 = local read "Touch lines"() -> (w160:T7)
                n271 = local read "DO Task"() -> (w156:refnum<k21>)
                n272 = local read "DI Task"() -> (w155:refnum<k21>)
                n273 = local read "Target"() -> (w162:i16)
                n274 = call "TargetCapture.vi"("DO Task"=w156, "Touch lines"=w160, "DI Task"=w155, "Home+target OK?"="Home+target OK?", "Target"=w162, "Initialize?"=w159) -> ("Go to stage"=w163:T8, "Last trial successful?"=w161:bool)  [unwired: 8 in]
                n275 = local write "Last trial successful?"(w161) -> ()
              }
              frame "Target hold init" {
                w169 = TRUE  # Initialize?
                n276 = local read "DO Task"() -> (w165:refnum<k21>)
                n277 = local read "DI Task"() -> (w164:refnum<k21>)
                n278 = local read "Target"() -> (w167:i16)
                n279 = call "TargetHold.vi"("DO Task"=w165, "DI Task"=w164, "target hold"="Hold duration", "target\nbounce-off"="Allowed\nbounce-off", "Target"=w167, "Post-capture brightness"="Post-capture brightness", "Initialize?"=w169) -> ()  [unwired: 7 in, 2 out]
              }
              frame "Target hold" {
                w176 = FALSE  # Initialize?
                n280 = local read "Home+target OK?"() -> (w174:bool)
                n281 = local read "Touch lines"() -> (w179:T7)
                n282 = local read "DO Task"() -> (w180:refnum<k21>)
                n283 = local read "DI Task"() -> (w173:refnum<k21>)
                n284 = local read "Target"() -> (w178:i16)
                n285 = call "TargetHold.vi"("DO Task"=w180, "Touch lines"=w179, "DI Task"=w173, "Home+target OK?"=w174, "Target"=w178, "Initialize?"=w176) -> ("Go to stage"=w181:T8, "Last trial successful?"=w177:bool)  [unwired: 8 in]
                n286 = local write "Last trial successful?"(w177) -> ()
              }
              frame "Reward stage" {
                # "This will be a bit written in the \ndata file so we're not worried about \nit reseting."
                n287 = Random Number (0-1)() -> (number: 0 to 1=w185:dbl)
                n288 = Multiply(x=w185, y=100.0) -> (x*y=w184:dbl)
                n289 = To Unsigned Long Integer(number=w184) -> (unsigned 32bit integer=w182:u32)
                n290 = Less Or Equal?(x=w182, y="Catch probability") -> (x <= y?=w187:bool)
                n291 = case shown="False" w187 {
                  selector: w187 -> [w194 w196]
                  tunnel: ["Reward duration" cluster{"Fix":dbl, "Rnd":dbl} {"Fix"=0.0, "Rnd"=0.0} ("Reward duration")] -> w192
                  tunnel: [w194 w196] -> w188
                  frame False {
                    # "Sending False bit for \ncatch trial"
                    # "Normal reward duration"
                  }
                  frame True {
                    # "Sending True bit for \ncatch trial"
                    # "This is the catch trial. \nSo we don't want to deliver \na reward"
                  }
                }
                "Catch Trial?" <- w188
                n292 = call "CalculateFixedPlusRandom2.vi"("Component times"=w192) -> ("time in ms"=w193:dbl)  [unwired: 1 in, 1 out]
                n293 = local read "DO Task"() -> (w189:refnum<k21>)
                n294 = call "Reward Pulse.vi"("Pulse duration (ms)"=w193, "DO Task"=w189) -> ()  [unwired: 8 in]
              }
              frame "Intertrial" {
                n295 = local read "Last trial successful?"() -> (w215:bool)
                n296 = local read "Bumps"() -> (w199:bool)
                n297 = local read "target set size"() -> (w203:i32)
                n298 = local read "# target sets"() -> (w204:u16)
                n299 = call "CalculateFixedPlusRandom2.vi"("Component times"="Intertrial interval") -> ("Composite time"=w216:dbl)  [unwired: 1 in, 1 out]
                n300 = local write "Override bumps"(w199) -> ()
                n301 = local write "Recenter motor"(w199) -> ()
                n302 = while {
                  shift-right: [enum16{"Start counting", "Read count", "Reset"}."Read count" ("Enum")] -> _
                  shift-left: enum16{"Start counting", "Read count", "Reset"}."Start counting" ("Enum") -> [w234]
                  tunnel: [w229] -> _
                  tunnel: w216 -> [w228]
                  stop <- w230 stop-if-true
                  n303 = call "non-Reentrant Controllable Timer.vi"("Enum"=w234) -> ("Time out"=w232:dbl)  [unwired: 1 in]
                  n304 = local read "stop"() -> (w231:bool)
                  n305 = Greater Or Equal?(x=w232, y=w228) -> (x >= y?=w229:bool)
                  n306 = Or(x=w229, y=w231) -> (x .or. y?=w230:bool)
                }
                n307 = Multiply(x=w204, y=w203) -> (x*y=w202:i32)
                n308 = call "TrackStats2.vi"("Last trial successful?"=w215, "Trial bin size"=w202, "Persistent\n Mode?"="Persistent\n Mode?", "Command"=enum16{"Reset", "Increment"}."Increment") -> ("Total incorrect"=→"Total incorrect":i32, "Total correct"=→"Total correct":i32, "# total trials"=→"Total trials":i32, "Total % correct"=w207:dbl, "Segment trials"=→"Block trials":i32, "Experiment trials"=→"Exp trials":i32, "Experiment correct"=→"Exp correct":i32, "Experiment %"=→"Exp %":dbl, "Segment Percentage"=w208:dbl)  [unwired: 3 in]
                "Block %" <- w208
                "Total %" <- w207
                n309 = Bundle("Segment Percentage"=w208, "Total % correct"=w207) -> (→"Waveform Chart":T6)  [unwired: 1 in]
                n310 = stacked-sequence {
                  frame #0 {
                    n311 = local read "Last trial successful?"() -> (w221:bool)
                    n312 = case shown="True" w221 {
                      frame False {
                        n313 = local read "DO Task"() -> (w222:refnum<k21>)
                        n314 = call "Signal Error.vi"("DO Task"=w222, "Error bong?"="Error\nbong?") -> ()  [unwired: 3 in]
                      }
                      frame True {
                      }
                    }
                  }
                  frame #1 {
                    n315 = local read "DO Task"() -> (w224:refnum<k21>)
                    n316 = call "WriteDigioBits2_DAQmx.vi"("Bits to write"=Bits_to_Write."In trial off", "DO Task"=w224) -> ()  [unwired: 9 in, 1 out]
                  }
                  frame #2 {
                  }
                }
                n317 = local read "Persistent\n Mode?"() -> (w205:bool)
                n318 = case shown="False" w205 {
                  tunnel: [w226 w227] -> w219
                  frame False {
                    w226 = TRUE  # End of trial
                  }
                  frame True {
                    n319 = local read "Last trial successful?"() -> (w227:bool)
                  }
                }
              }
            }
            n320 = Wait (ms)(milliseconds to wait=u32 1) -> ()  [unwired: 1 out]
            n321 = Compound Arithmetic op=OR(w63, "stop") -> (w61:bool)
            "Current stage" <- w65
          }
          n322 = local read "Exp reset"() -> (w51:bool)
          n323 = Compound Arithmetic op=OR(w53, w52, w51) -> (w50:bool)
        }
        n324 = Or(x=w48, y=w47) -> (x .or. y?=w46:bool)
      }
    }
    frame #3 {
      # "Turn LED's, \nbuzzer,\npump off\njust to be\nsure"
      n325 = local read "DO Task"() -> (w407:refnum<k21>)
      n326 = local read "DO Task"() -> (w405:refnum<k21>)
      n327 = local read "DO Task"() -> (w409:refnum<k21>)
      n328 = local read "DO Task"() -> (w410:refnum<k21>)
      n329 = local read "DO Task"() -> (w412:refnum<k21>)
      n330 = local read "DO Task"() -> (w414:refnum<k21>)
      n331 = local write "Record flag"(FALSE ("Record flag")) -> ()
      n332 = call "WriteDigioBits2_DAQmx.vi"("Bits to write"=Bits_to_Write."In trial off", "DO Task"=w407) -> ()  [unwired: 9 in, 1 out]
      n333 = call "WriteDigioBits2_DAQmx.vi"("Bits to write"=Bits_to_Write."All LEDs off", "DO Task"=w405) -> ()  [unwired: 9 in, 1 out]
      n334 = call "WriteDigioBits2_DAQmx.vi"("Bits to write"=Bits_to_Write."Buzzer off", "DO Task"=w409) -> ()  [unwired: 9 in, 1 out]
      n335 = call "WriteDigioBits2_DAQmx.vi"("Bits to write"=Bits_to_Write."Reward off", "DO Task"=w410) -> ()  [unwired: 9 in, 1 out]
      n336 = call "WriteDigioBits2_DAQmx.vi"("Bits to write"=Bits_to_Write."Error off", "DO Task"=w412) -> ()  [unwired: 9 in, 1 out]
      n337 = call "WriteDigioBits2_DAQmx.vi"("Bits to write"=Bits_to_Write."DBS off", "DO Task"=w414) -> ()  [unwired: 9 in, 1 out]
      n338 = local write "stop"(FALSE ("stop")) -> ()
    }
  }
